vi "PE_DataAcquisition.vi"() -> ()   [LabVIEW 2016]
uses:
  database/database.lvlib
  <vilib>/Instr/_visa.llb/VISA Configure Serial Port (Instr).vi
  SerialSupport/Serial - Settings.ctl
  SerialSupport/Serial - ASCII Characters.ctl
  SerialSupport/Serial - XON-XOFF Characters.ctl
panel:
  out "CtrlCmdMsg 2":string
  out "当前指令 2":string
  in  "标记 2":dbl
  in  "TestId 2":string
  out "CtrlCmdMsg":string
  out "串口信息发送持久化":bool=TRUE
  out "串口信息发送":bool=TRUE
  out "UDP发送持久化":bool=TRUE
  out "TCP发送持久化":bool=TRUE
  out "串口接收持久化":bool=TRUE
  in  "串口发送按钮":bool
  in  "Serial output":string caption="字符串输出"
  in  "终止符":u8=10 format="%.0x"
  in  "终止符时结束写入？":bool=TRUE
  in  "VISA资源名称":refnum<visa-resource-name>="COM10"
  in  "XON/XOFF字符":T1={"XON"=enum."DC1", "XOFF"=enum."DC3"}
  in  "串口设置":T3={"波特率"=115200, "数据位"=8, "校验"=enum."None", "停止位"=10, "流控制"=0} {"流控制" items=["无"=0, "XON/XOFF"=1, "RTS/CTS"=2, "DTR/DSR"=4]; "停止位" items=["1.0"=10, "1.5"=15, "2.0"=20]; "数据位" min=5 max=8 step=1; "波特率" items=["75"=75, "110"=110, "134"=134, "150"=150, "300"=300, "600"=600, "1200"=1200, "1800"=1800, "2400"=2400, "4800"=4800, "7200"=7200, "9600"=9600, "14400"=14400, "19200"=19200, "28800"=28800, "38400"=38400, "56000"=56000, "57600"=57600, "115200"=115200, "128000"=128000, "230400"=230400]}
  in  "终止符时结束读取？":bool=TRUE
  in  "读取":bool=TRUE
  in  "串口停止":bool
  in  "串口发送命令":string="{\"cmd\":\"CT_ON\",\"id\":\"C_FR\",on:true}"
  out "串口信息":string
  in  "串口最大字节":u32=1000
  out "当前指令":string
  in  "错误输入 16":errorcluster caption="错误输入"
  in  "TestId":string
  in  "dataLabel":string
  in  "总状态":string
  in  "msgid":dbl
  # "用于说明数据来源等 如串口"
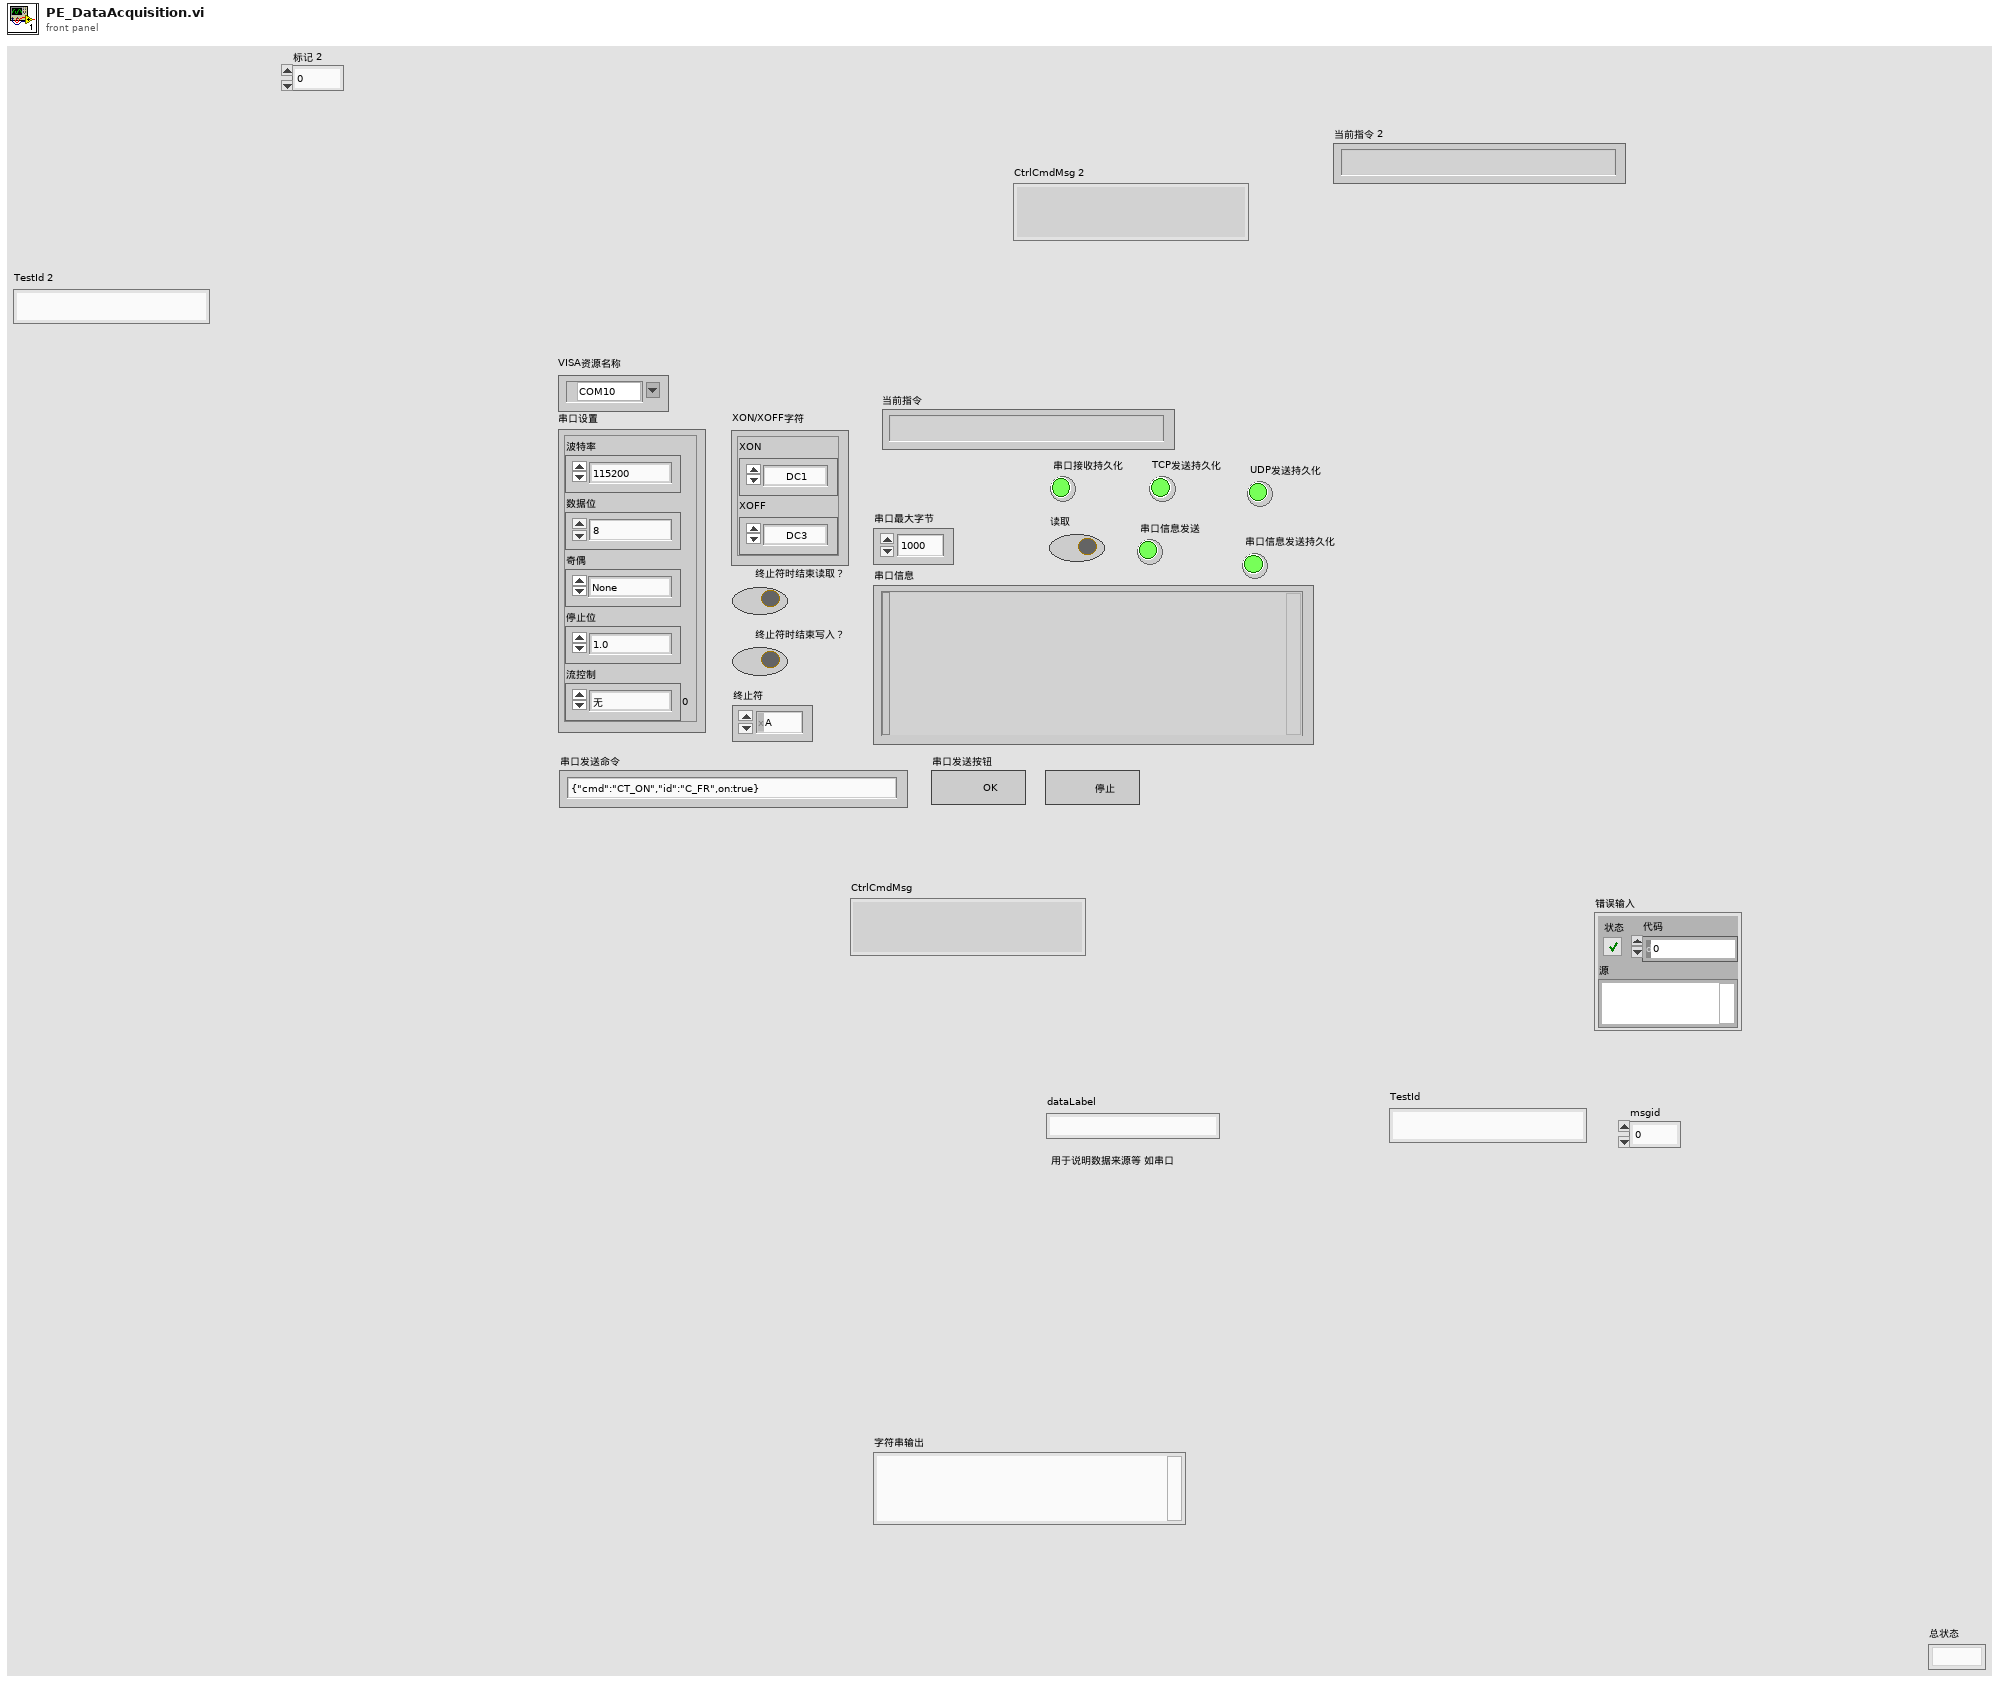
[diagram p1: front panel]
types:
  T1 = typedef "Serial - XON-XOFF Characters.ctl" = cluster{"XON":T2, "XOFF":T2}
  T2 = typedef "Serial - ASCII Characters.ctl" = enum16{"NUL", "SOH", "STX", "ETX", "EOT", "ENQ", "ACK", "BEL", "BS", "HT", "LF", "VT", "FF", "CR", "SO", "SI", "DLE", "DC1", "DC2", "DC3", "DC4", "NAK", "SYN", "ETB", "CAN", "EM", "SUB", "ESC", "FS", "GS", "RS", "US", "SP", "!", "\"", "#", "$", "%", "&", "'", "(", ")", "*", "+", ",", "- (-)", ".", "/", "0", "1", "2", "3", "4", "5", "6", "7", "8", "9", ":", ";", "<", "=", ">", "?", "@", "A", "B", "C", "D", "E", "F", "G", "H", "I", "J", "K", "L", "M", "N", "O", "P", "Q", "R", "S", "T", "U", "V", "W", "X", "Y", "Z", "[", "\\", "]", "^", "_", "`", "a", "b", "c", "d", "e", "f", "g", "h", "i", "j", "k", "l", "m", "n", "o", "p", "q", "r", "s", "t", "u", "v", "w", "x", "y", "z", "{", "|", "}", "~"}
  T3 = typedef "Serial - Settings.ctl" = cluster{"波特率":u32, "数据位":u16, "校验":enum16{"None", "Odd", "Even", "Mark", "Space"}, "停止位":u16, "流控制":u16}
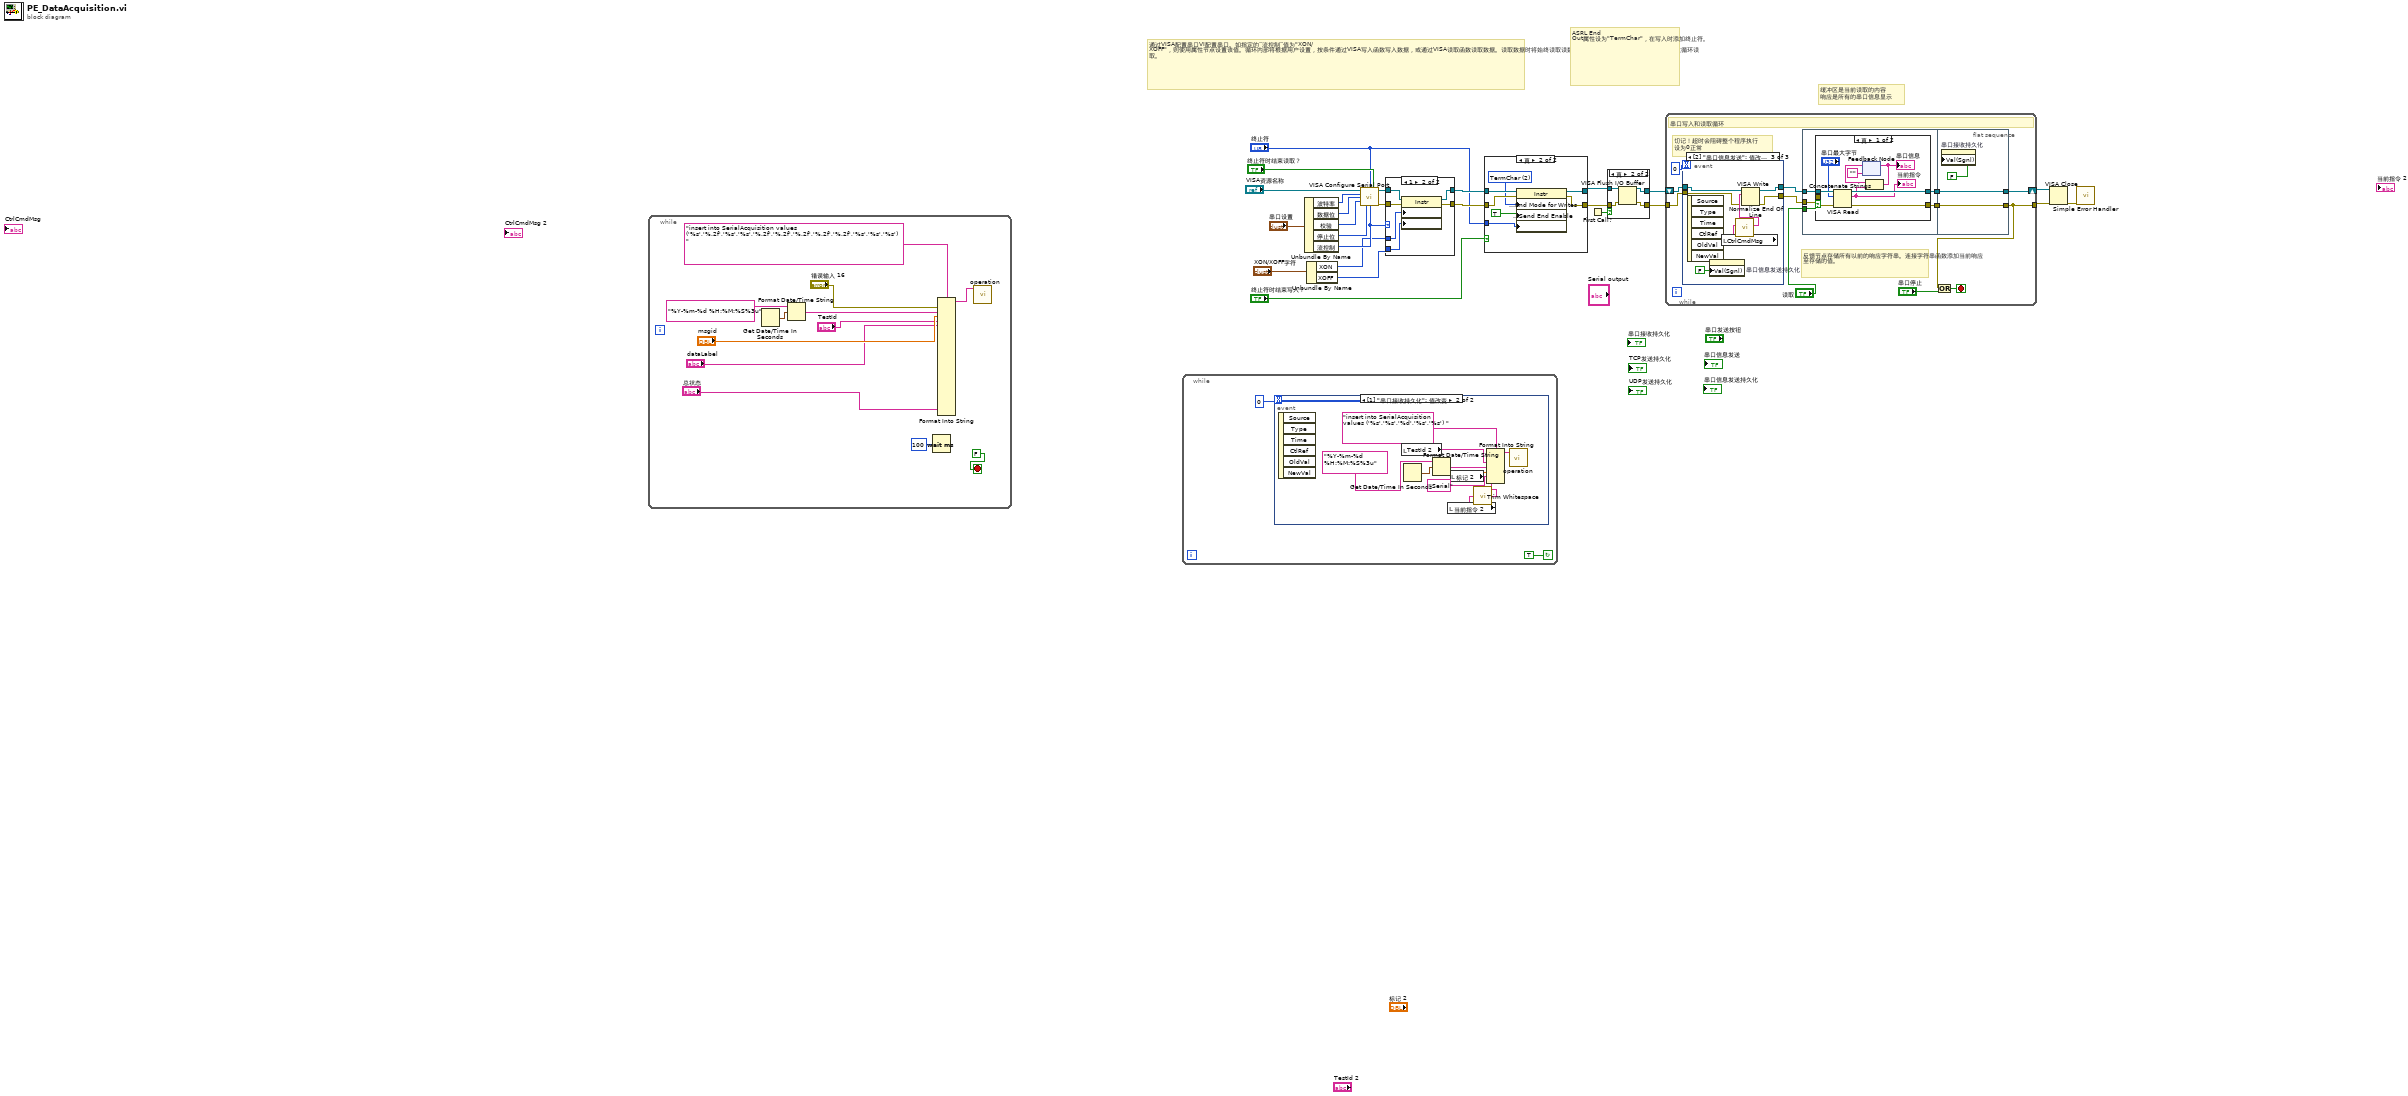
[diagram p0: block diagram]
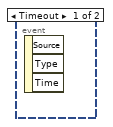
[diagram p2: hidden frame]
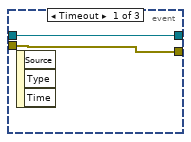
[diagram p7: hidden frame]
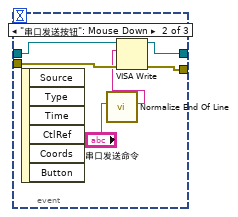
[diagram p8: hidden frame]
diagram:
  # "缓冲区是当前读取的内容\n响应是所有的串口信息显示"
  # "ASRL End Out属性设为\"TermChar\"，在写入时添加终止符。"
  # "通过VISA配置串口VI配置串口。如指定的“流控制”值为\"XON/XOFF\"，则使用属性节点设置该值。循环内部将根据用户设置，按条件通过VISA写入函数写入数据，或通过VISA读取函数读取数据。读取数据时将始终读取读数值指定的数据数量。多余数据将在下一次循环读取。"
  n1 = while {
    stop <- FALSE stop-if-true
    n2 = Get Date/Time In Seconds() -> (seconds since 1Jan1904=w33:timestamp)
    n3 = Format Date/Time String ("格式化日期/时间字符串")(time format string (%c)="%Y-%m-%d %H:%M:%S%3u" ("时间格式字符串(%c)"), seconds (now)=w33) -> (date/time string=w29:string)  [unwired: 1 in]
    n4 = Wait (ms)(milliseconds to wait=u32 100) -> ()  [unwired: 1 out]
    n5 = Format Into String(format string="insert into SerialAcquisition values ('%s','%.2f','%s','%s','%.2f','%.2f','%.2f','%.2f','%.2f','%s','%s','%s')                                                                " ("格式字符串"), error in="错误输入 16", w29, "msgid", "TestId", "dataLabel", "总状态") -> (resulting string=w36:string)  [unwired: 19 in, 1 out]
    n6 = call "operation.vi"("Command Text"=w36) -> ()  [unwired: 9 in, 1 out]
  }
  n7 = while {
    stop <- TRUE continue-if-true
    n8 = event shown="[1] \"串口接收持久化\": 值改变" {
      selector: _ -> [_ _]
      dyn-events: _ -> [_ _]
      timeout: 0 -> [_ _]
      event Timeout {
        n9 = event-data() -> ()  [unwired: 1 in, 3 out]
      }
      event "串口接收持久化": Value Change {
        n10 = event-data() -> ()  [unwired: 1 in, 6 out]
        n11 = local read "TestId 2"() -> (w45:string)
        n12 = Get Date/Time In Seconds() -> (seconds since 1Jan1904=w46:timestamp)
        n13 = Format Date/Time String ("格式化日期/时间字符串")(time format string (%c)="%Y-%m-%d %H:%M:%S%3u" ("时间格式字符串(%c)"), seconds (now)=w46) -> (date/time string=w47:string)  [unwired: 1 in]
        n14 = local read "当前指令 2"() -> (w42:string)
        n15 = local read "标记 2"() -> (w48:dbl)
        n16 = call <vilib>:"Trim Whitespace.vi"("string"=w42) -> ("trimmed string"=w41:string)  [unwired: 1 in]
        n17 = Format Into String(format string="insert into SerialAcquisition values ('%s','%s','%d','%s','%s') " ("格式字符串"), w45, w47, w48, "Serial" ("input 4"), w41) -> (resulting string=w44:string)  [unwired: 2 in, 1 out]
        n18 = call "operation.vi"("Command Text"=w44) -> ()  [unwired: 9 in, 1 out]
      }
    }
  }
  n19 = Unbundle By Name("串口设置") -> ("波特率"=w18:u32, "数据位"=w19:u16, "校验"=w20:enum16{"None", "Odd", "Even", "Mark", "Space"}, "停止位"=w21:u16, "流控制"=w12:u16)
  n20 = Unbundle By Name("XON/XOFF字符") -> ("XON"=w11:T2, "XOFF"=w10:T2)
  n21 = call-poly "VISA Configure Serial Port"("VISA resource name"="VISA资源名称", "termination char\n(0xA = '\\n' = LF)"="终止符", "Enable Termination\nChar (T)"="终止符时结束读取？", "baud rate (9600)"=w18, "data bits (8)"=w19, "parity (0:none)"=w20, "stop bits (10: 1 bit)"=w21, "flow control (0:none)"=w12) -> ("VISA resource name out"=w22:refnum<visa-resource-name>, "error out"=w23:errorcluster)  [unwired: 2 in, 4 out]
  n22 = case shown="1" w12 {
    tunnel: [w50 w57] -> w9
    tunnel: [w51 w56] -> w8
    tunnel: w23 -> [w50 w55]
    tunnel: w22 -> [w51 w54]
    tunnel: w11 -> [_ w53]
    tunnel: w10 -> [_ w52]
    frame Default {
    }
    frame 1 {
      n23 = property class="Instr"(reference=w54, error in=w55, "Serial Settings:Flow Control XON Character"=w53, "Serial Settings:Flow Control XOFF Character"=w52) -> (reference out=w56:refnum<visa-resource-name>, error out=w57:errorcluster)
    }
  }
  n24 = case shown="真" "终止符时结束写入？" {
    tunnel: w8 -> [w58 w66]
    tunnel: w9 -> [w59 w65]
    tunnel: [w58 w64] -> w5
    tunnel: [w59 w63] -> w4
    tunnel: "终止符" -> [_ w61]
    frame False {
    }
    frame True {
      w62 = u16 2 items=["None", "LastBit", "TermChar", "Break"] ("Serial Settings:Serial End Mode for Writes")
      n25 = property class="Instr"(reference=w66, error in=w65, "Serial Settings:End Mode for Writes"=w62, "Message Based Settings:Send End Enable"=TRUE, "Message Based Settings:Termination Character"=w61) -> (reference out=w64:refnum<visa-resource-name>, error out=w63:errorcluster)
    }
  }
  n26 = First Call?() -> (First Call?: T/F=w1:bool)
  n27 = case shown="真" w1 {
    tunnel: w5 -> [w68 w72]
    tunnel: w4 -> [w67 w71]
    tunnel: [w68 w70] -> w3
    tunnel: [w67 w69] -> w2
    frame False {
    }
    frame True {
      n28 = VISA Flush I/O Buffer(VISA resource name=w72, error in (no error)=w71) -> (VISA resource name out=w70:refnum<visa-resource-name>, error out=w69:errorcluster)  [unwired: 1 in]
    }
  }
  n29 = while {
    shift-right: [w84] -> w13
    shift-left: w3 -> [w77]
    tunnel: w2 -> [w79]
    tunnel: [w81] -> w14
    stop <- w82 stop-if-true
    # "反馈节点存储所有以前的响应字符串。连接字符串函数添加当前响应至存储的值。"
    # "切记！超时会阻碍整个程序执行\n设为0正常"
    # "串口写入和读取循环"
    n30 = event shown="[2] \"串口信息发送\": 值改变" {
      selector: _ -> [_ _ _]
      dyn-events: _ -> [_ _ _]
      timeout: 0 -> [_ _ _]
      tunnel: w79 -> [w104 w111 w114]
      tunnel: [w104 w110 w115] -> w78
      tunnel: w77 -> [w105 w109 w117]
      tunnel: [w105 w108 w116] -> w76
      event Timeout {
        n31 = event-data() -> ()  [unwired: 1 in, 3 out]
      }
      event "串口发送按钮": Mouse Down {
        n32 = event-data() -> ()  [unwired: 1 in, 6 out]
        n33 = call <vilib>:"Normalize End Of Line.vi"("string in"="串口发送命令") -> ("string out"=w106:string)  [unwired: 7 in]
        n34 = VISA Write(VISA resource name=w109, write buffer=w106, error in (no error)=w111) -> (VISA resource name out=w108:refnum<visa-resource-name>, error out=w110:errorcluster)  [unwired: 1 out]
      }
      event "串口信息发送": Value Change {
        n35 = event-data() -> ()  [unwired: 1 in, 6 out]
        n36 = property on="串口信息发送持久化" class="Bool (严格)"("Val(Sgnl)"=FALSE ("Value (Signaling)")) -> ()  [unwired: 2 in, 2 out]
        n37 = local read "CtrlCmdMsg"() -> (w113:string)
        n38 = call <vilib>:"Normalize End Of Line.vi"("string in"=w113) -> ("string out"=w118:string)  [unwired: 7 in]
        n39 = VISA Write(VISA resource name=w117, write buffer=w118, error in (no error)=w114) -> (VISA resource name out=w116:refnum<visa-resource-name>, error out=w115:errorcluster)  [unwired: 1 out]
      }
    }
    n40 = flat-sequence {
      tunnel: "读取" -> [w88]
      tunnel: w78 -> [w86]
      tunnel: w76 -> [w85]
      tunnel: [w89] -> w74
      tunnel: [w87] -> w73
      tunnel: [w102] -> w81
      tunnel: [w103] -> w84
      tunnel: w74 -> [w103]
      tunnel: w73 -> [w102]
      frame #0 {
        n41 = case shown="真" w88 {
          tunnel: [w96 w100] -> w89
          tunnel: w85 -> [w98 w100]
          tunnel: [w94 w99] -> w87
          tunnel: w86 -> [w97 w99]
          frame True {
            n42 = VISA Read(VISA resource name=w98, byte count="串口最大字节", error in (no error)=w97) -> (VISA resource name out=w96:refnum<visa-resource-name>, read buffer=w90:string, error out=w94:errorcluster)  [unwired: 1 out]
            "当前指令" <- w90
            n43 = feedback #1("") -> (w93:string)
            n44 = Concatenate Strings(w93, w90) -> (w92:string)
            "串口信息" <- w92
            n45 = feedback-in #1(w92) -> ()
          }
          frame False {
          }
        }
      }
      frame #1 {
        n46 = property on="串口接收持久化" class="Bool (严格)"("Val(Sgnl)"=FALSE ("Value (Signaling)")) -> ()  [unwired: 2 in, 2 out]
      }
    }
    n47 = Or(x=w81, y="串口停止") -> (x .or. y?=w82:bool)
  }
  n48 = VISA Close(VISA resource name=w13, error in (no error)=w14) -> (error out=w15:errorcluster)
  n49 = call <vilib>:"Simple Error Handler.vi"("error in (no error)"=w15) -> ()  [unwired: 1 in, 8 out]
